vi "lvcsm Read section As StringList.vi"(6 "Config Path (\"\" For Lvcsm File)":path, 8 "error in (no error)":errorcluster, 10 "API Name":string="CSMAPI", 11 "CSM Name":string) -> (0 "error out":errorcluster, 3 "CSMAPI List":string[](array[string]))   [LabVIEW 2017, in "lvcsm File Support.lvlib"]
uses:
  lvcsm File Support.lvlib
  b7efc127-9b6c-49b9-9e9d-39643bcb625b.vi
  d58331e6-8071-4439-9abb-a72bbe2c8ea8.vi
  _Array of VData to VCluster.vi
  <vilib>/Utility/config.llb/Close Config Data.vi
  <vilib>/Utility/config.llb/Read Key.vi
  <vilib>/Utility/config.llb/Read Key (Double).vi
  <vilib>/Utility/config.llb/Read Key (I32).vi
  lvcsm String to Path.vi
  <vilib>/Utility/config.llb/Read Key (String).vi
  Path to lvcsm String.vi
  <vilib>/Utility/config.llb/Get Key Names.vi
  <vilib>/Utility/Data Type/Get Type Information.vi
  <vilib>/Utility/Data Type/Get Array Information.vi
  <vilib>/Utility/config.llb/Read Key (Boolean).vi
  <vilib>/Utility/config.llb/Open Config Data.vi
  lvcsm File Path.vi
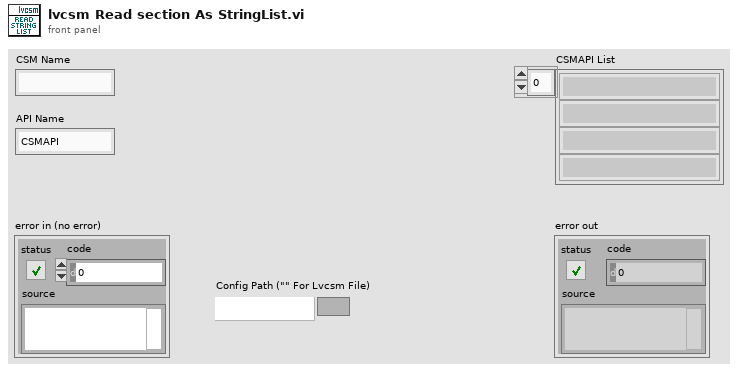
[diagram p1: front panel]
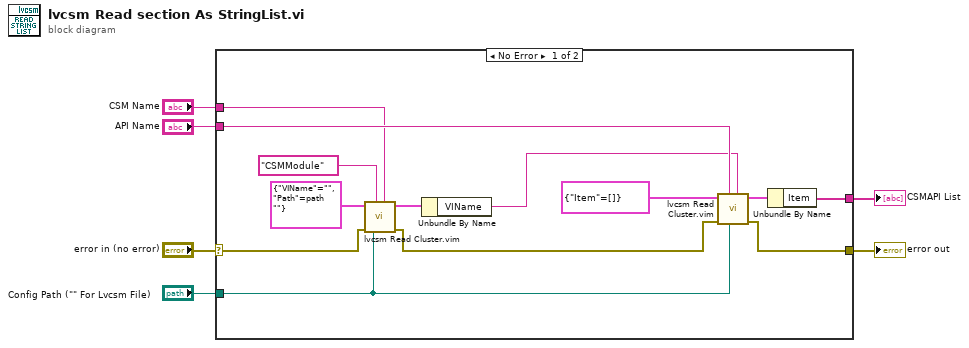
[diagram p0: block diagram]
diagram:
  n1 = case shown="No Error" "error in (no error)" {
    selector: "error in (no error)" -> [w10 w20]
    tunnel: [w16 w20] -> w6
    tunnel: "CSM Name" -> [w12 _]
    tunnel: [w17 _] -> w3
    tunnel: "Config Path (\"\" For Lvcsm File)" -> [w11 _]
    tunnel: "API Name" -> [w15 _]
    frame No Error {
      n2 = call "lvcsm Read Cluster.vim"("Sub-section (\"\")"=w12, "Config Path"=w11, "Section"="CSMModule", "Error In"=w10, "Default Prototype"=cluster{"VIName":string, "Path":path} {"VIName"="", "Path"=path ""}) -> ("error out"=w9:errorcluster, "Cluster (Dup)"=w8:cluster{"VIName":string, "Path":path})  [unwired: 5 in]
      n3 = Unbundle By Name(w8) -> ("VIName"=w7:string)
      n4 = call "lvcsm Read Cluster.vim"("Sub-section (\"\")"=w7, "Config Path"=w11, "Section"=w15, "Error In"=w9, "Default Prototype"=cluster{"Item":string[]} {"Item"=[]}) -> ("error out"=w16:errorcluster, "Cluster (Dup)"=w19:cluster{"Item":string[]})  [unwired: 5 in]
      n5 = Unbundle By Name(w19) -> ("Item"=w17:string[])
    }
    frame Error {
    }
  }
  "error out" <- w6
  "CSMAPI List" <- w3
